vi "Key and Value Strings to JSON Row.vi"(10 "Value":string="3", 11 "Key":string="Wonder") -> (3 "resulting string":string)   [LabVIEW 2011]
uses:
  <vilib>/regexp/Match Regular Expression.xnode
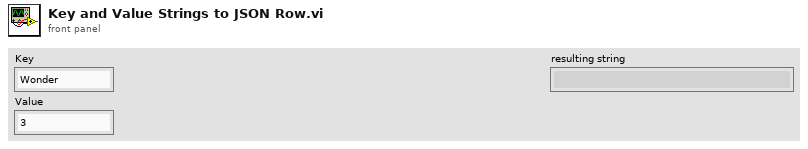
[diagram p1: front panel]
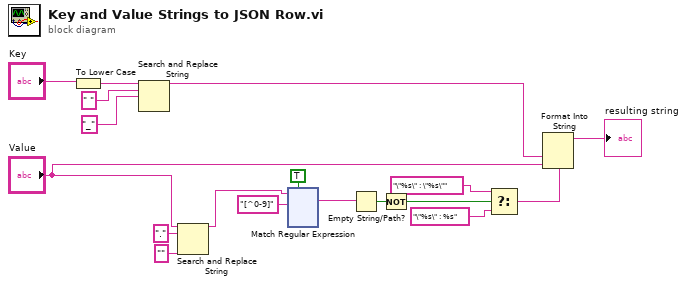
[diagram p0: block diagram]
diagram:
  n1 = To Lower Case(string="Key") -> (all lower case string=w12:string)
  n2 = Search and Replace String(input string=w12, search string=" ", replace string="_" ("replace string (\"\")")) -> (result string=w9:string)  [unwired: 5 in, 3 out]
  n3 = Search and Replace String(input string="Value", search string=".", replace string="" ("replace string (\"\")")) -> (result string=w3:string)  [unwired: 5 in, 3 out]
  n4 = xnode "Match Regular Expression"("input string"=w3, "regular expression"="[^0-9]", "ignore case? (F)"=TRUE) -> ("whole match"=w17:string)  [unwired: 3 in, 4 out]
  n5 = Empty String/Path?(string/path=w17) -> (empty?=w16:bool)
  n6 = Not(x=w16) -> (.not. x?=w2:bool)
  n7 = Select(t="\"%s\" : \"%s\"" ("format string"), s=w2, f="\"%s\" : %s" ("format string")) -> (s? t:f=w15:string)
  n8 = Format Into String(format string=w15, w9, "Value") -> (resulting string=→"resulting string":string)  [unwired: 2 in, 1 out]
